vi "Unmarshal.vi"(8 "error in (no error)":errorcluster, 10 "Buffer":u8[](array[numeric]), 11 "Tag in":refnum<class "Basic Type.lvclass">) -> (0 "error out":errorcluster, 2 "Buffer Count":i32, 3 "Tag out":refnum<class "Basic Type.lvclass">)   [LabVIEW 2020, in "Protobuf RAW.lvlib" / "Basic Type.lvclass"]
uses:
  Basic Type.lvclass
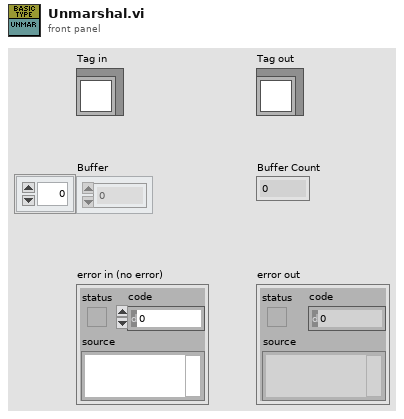
[diagram p1: front panel]
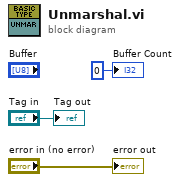
[diagram p0: block diagram]
diagram:
  "error out" <- "error in (no error)"
  "Tag out" <- "Tag in"
  "Buffer Count" <- 0
